vi "Wärmepumpe.ParameterUI.vi"() -> ()   [LabVIEW 2016, in "Wärmepumpe.lvclass"]
uses:
  Package ResourceControl/ViHandler/ViHandler.ViInfo.ctl
  Package Libraries/Message Queue/private/MessageQueue.MessageTypeDef.ctl
  Package ErrorHandling/ErrorHandling.lvclass/ErrorHandling.ctl
  Package ErrorHandling/ErrorHandling.checkForErrorAndHandle.vi
  Package ErrorHandling/ErrorHandling.GetErrorHandler.vi
  Package Libraries/StringFunctions/StringFunctions_ReplaceAllBlindSigns.vi
  <vilib>/dlg_ctls.llb/Space Constant.vi
  <vilib>/Utility/error.llb/Error Cluster From Error Code.vi
  Package Libraries/TimingFunctions/TimingFunctions_getUtcTimestamp.vi
  <vilib>/Utility/error.llb/Trim Whitespace.vi
  <vilib>/Utility/error.llb/Search and Replace Pattern.vi
  Package ErrorHandling/ErrorHandling.addLastErrorToFile.vi
  <vilib>/ErrorRing/Error Ring.xnode
  Package ErrorHandling/ErrorHandling.lvclass
  Package ResourceControl/ViHandler/ViHandler.lvclass
panel:
  in  "Wärmepumpe Parameter":T1
  out "Y-AxisCopy":dbl[](array[numeric])=[54400.0, 48000.0, 40000.0, 30000.0] caption="Y-Axis"
  out "X-AxisCopy":dbl[](array[numeric])=[54400.0, 48000.0, 40000.0, 30000.0] caption="X-Axis"
  in  "Heizleistung":dbl[][](array[numeric])=[[54400.0, 48000.0, 40000.0, 30000.0], [65800.0, 58800.0, 52800.0, 45000.0], [78600.0, 70400.0, 63800.0, 58200.0], [92400.0, 83200.0, 76400.0, 71400.0], [108800.0, 98000.0, 89800.0, 82200.0], [126800.0, 114600.0, 105200.0, 98400.0]]
  out "Y-Axis":dbl[](array[numeric])=[54400.0, 48000.0, 40000.0, 30000.0]
  out "X-Axis":dbl[](array[numeric])=[54400.0, 48000.0, 40000.0, 30000.0]
  in  "Kältelteistung":dbl[][](array[numeric])=[[54400.0, 48000.0, 40000.0, 30000.0], [65800.0, 58800.0, 52800.0, 45000.0], [78600.0, 70400.0, 63800.0, 58200.0], [92400.0, 83200.0, 76400.0, 71400.0], [108800.0, 98000.0, 89800.0, 82200.0], [126800.0, 114600.0, 105200.0, 98400.0]]
  in  "LoadDefBtn":bool
  in  "Model Path":path
  out "Wärmepumpe":refnum<data-value>
  out "ViInfoTemp":T2
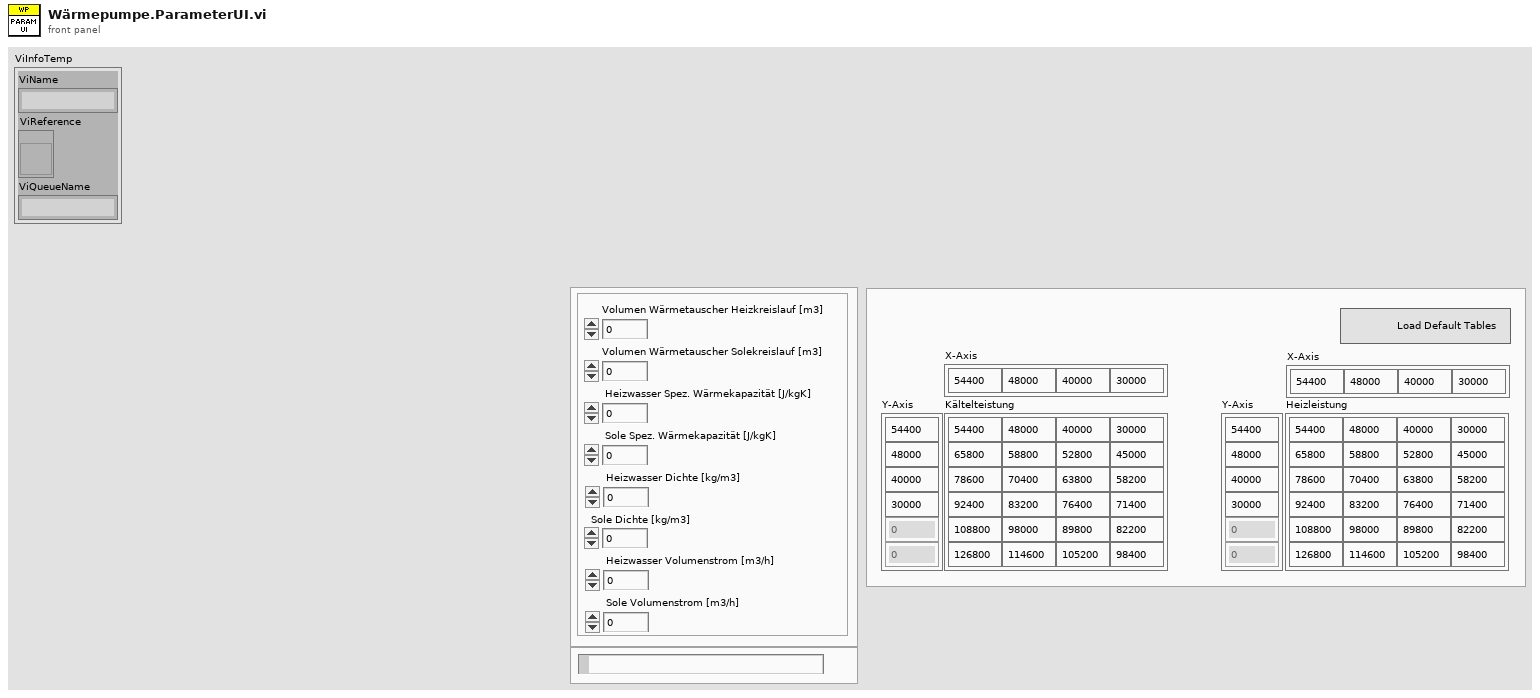
[diagram p1: front panel]
types:
  T1 = cluster{"Volumen Wärmetauscher Heizkreislauf [m3]":dbl, "Volumen Wärmetauscher Solekreislauf [m3]":dbl, " Heizwasser Spez. Wärmekapazität [J/kgK]":dbl, " Sole Spez. Wärmekapazität [J/kgK]":dbl, " Heizwasser Dichte [kg/m3]":dbl, "Sole Dichte [kg/m3] ":dbl, " Heizwasser Volumenstrom [m3/h]":dbl, " Sole Volumenstrom [m3/h]":dbl}
  T2 = typedef "ViHandler.lvclass/ViHandler.ViInfo.ctl" = cluster{"ViName":string, "ViReference":refnum<vi>, "ViQueueName":string}
  T3 = typedef "MessageQueue.MessageTypeDef.ctl" = cluster{"Message":string, "Data":variant}
  T4 = enum16{"open", "replace", "create", "open or create", "replace or create", "replace or create with confirmation"}
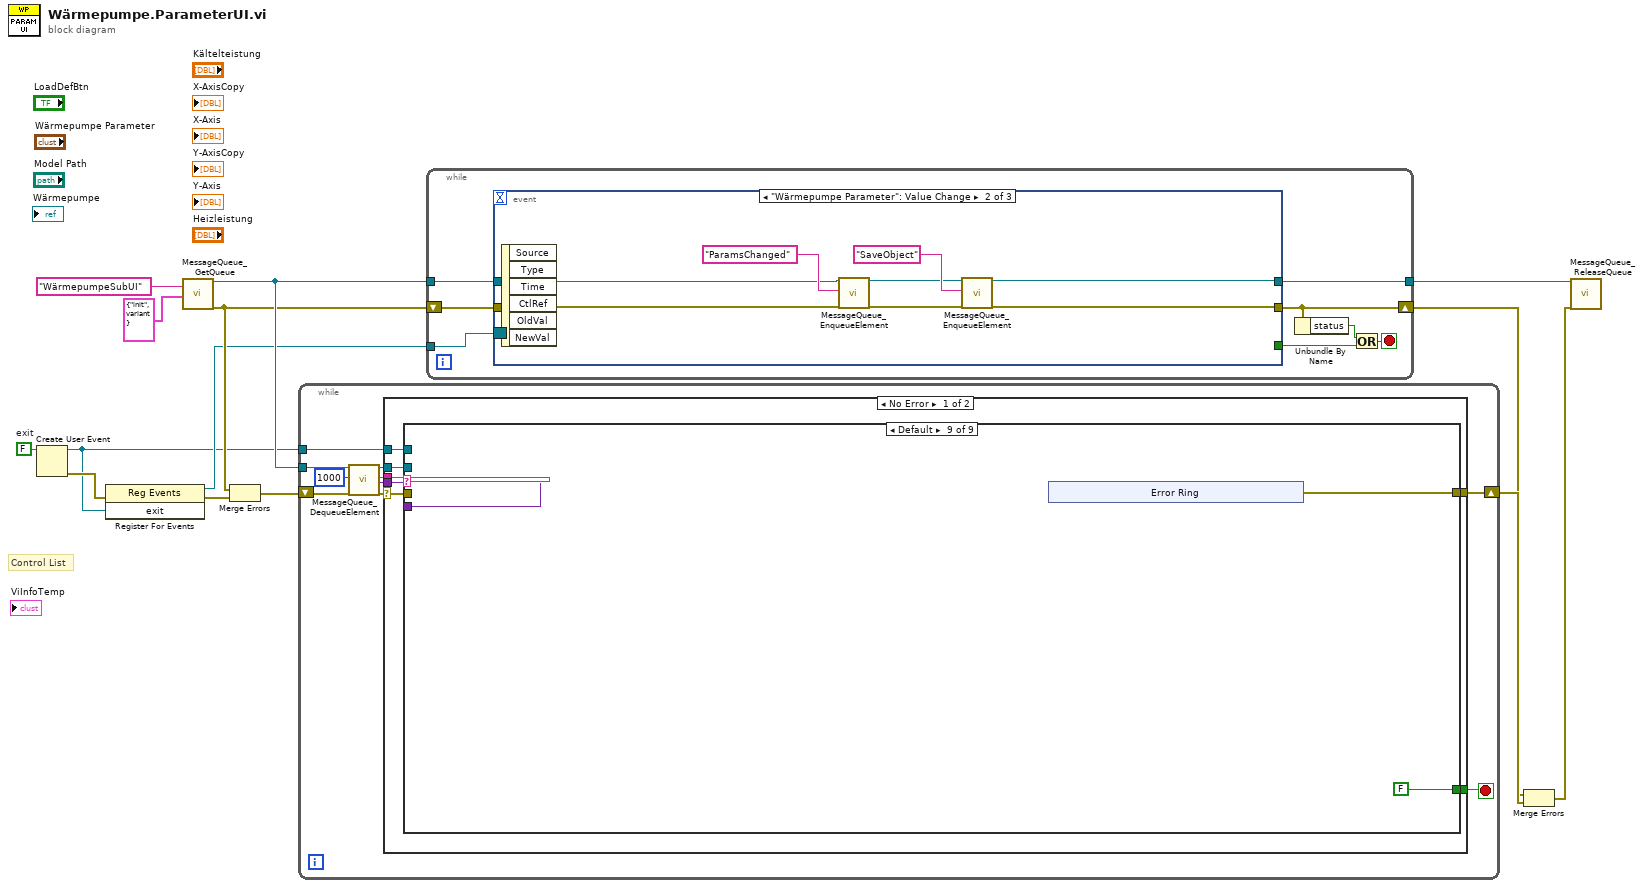
[diagram p0: block diagram]
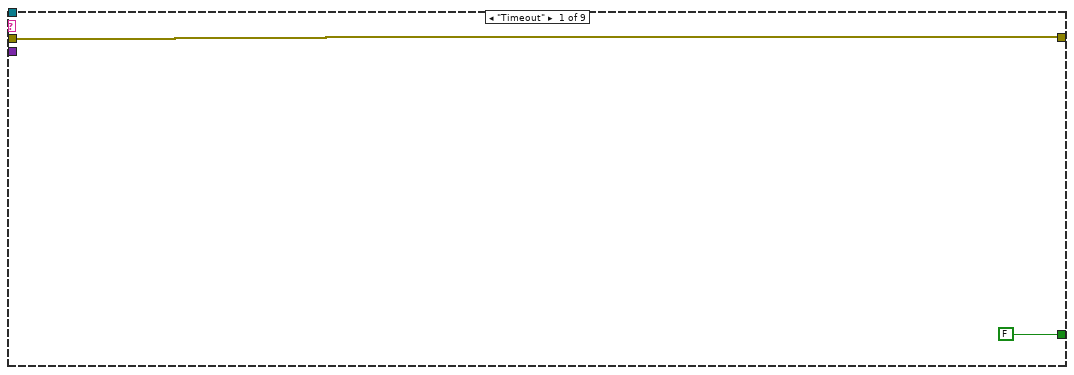
[diagram p2: hidden frame]
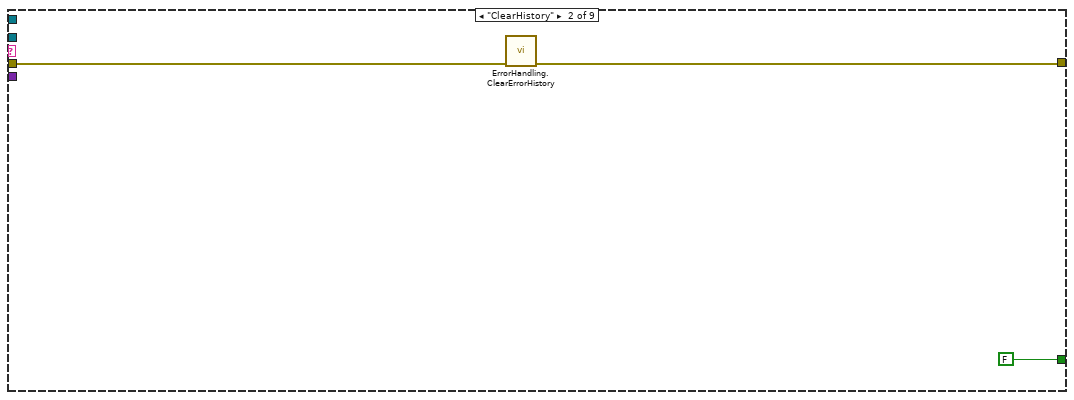
[diagram p3: hidden frame]
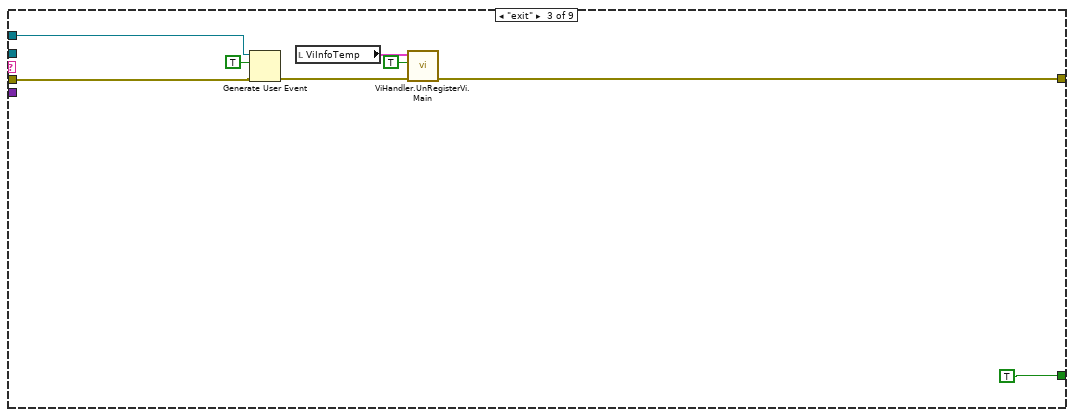
[diagram p4: hidden frame]
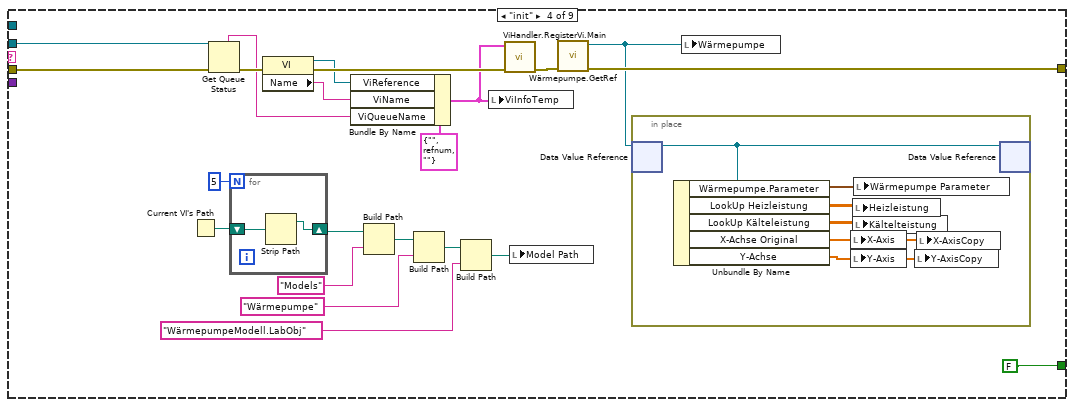
[diagram p5: hidden frame]
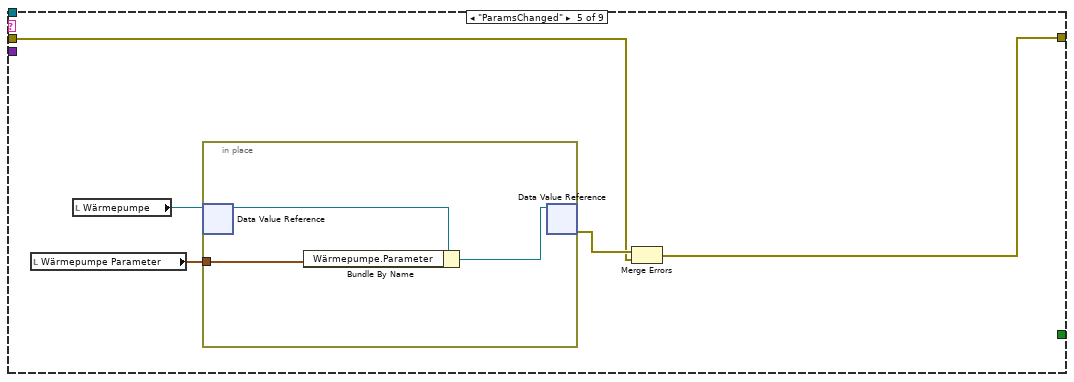
[diagram p6: hidden frame]
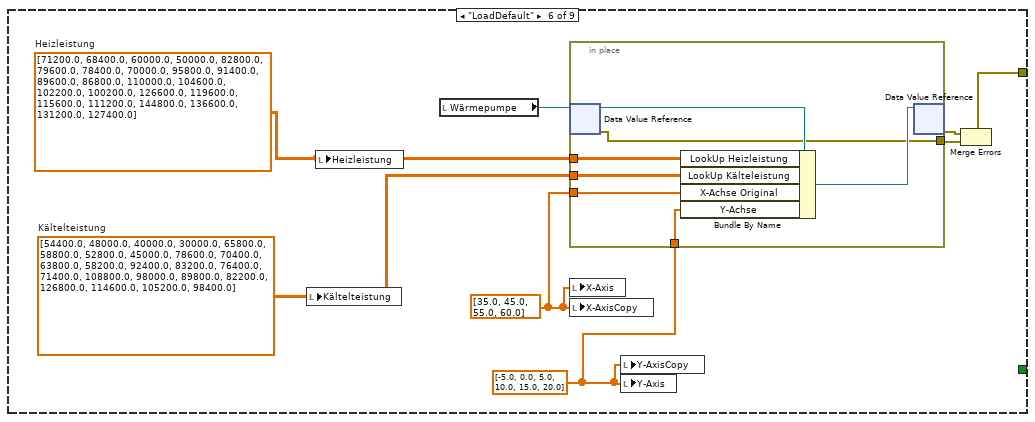
[diagram p7: hidden frame]
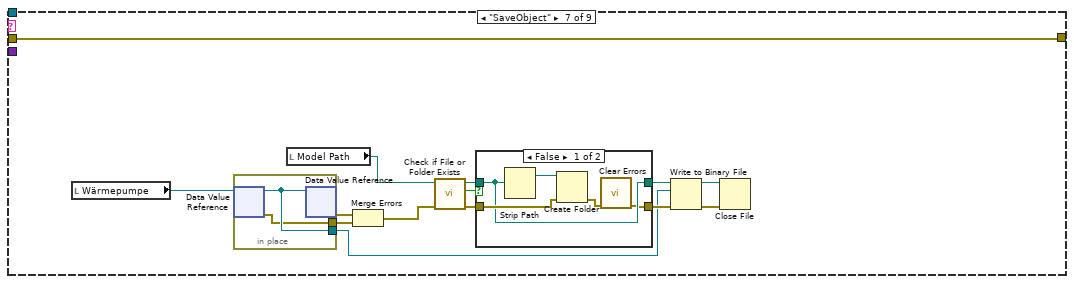
[diagram p8: hidden frame]
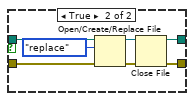
[diagram p9: hidden frame]
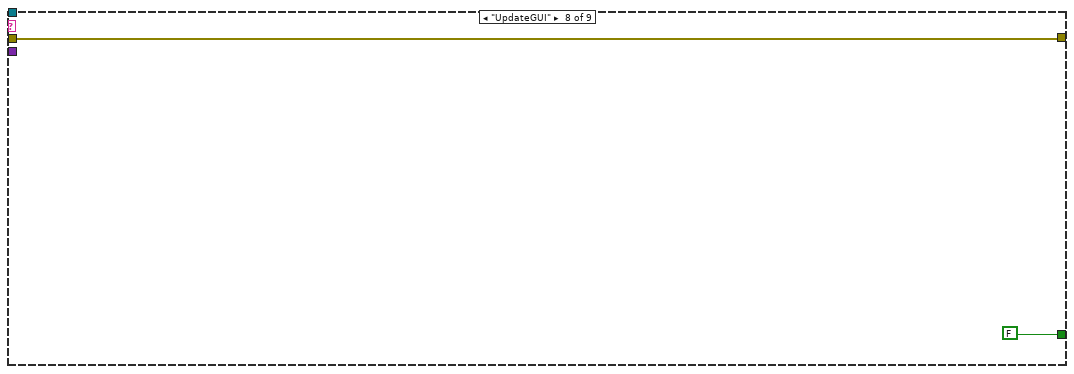
[diagram p10: hidden frame]
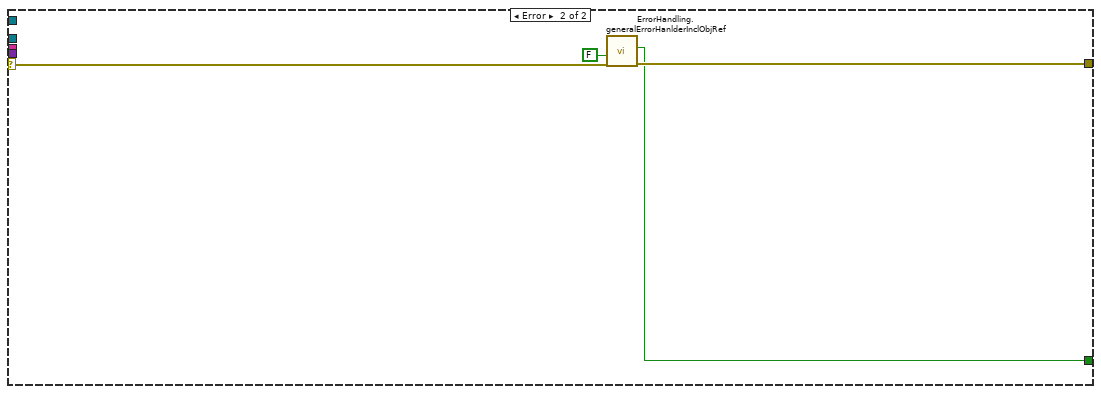
[diagram p11: hidden frame]
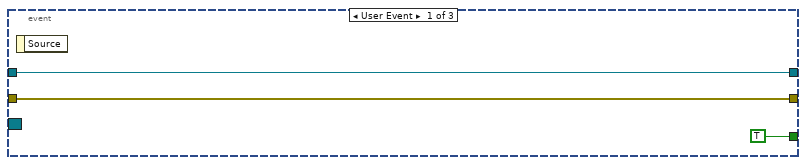
[diagram p12: hidden frame]
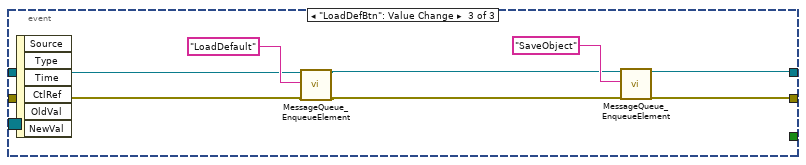
[diagram p13: hidden frame]
diagram:
  w7 = FALSE  # exit
  # "Control List"
  n1 = Create User Event(user event datatype=w7) -> (user event=w5:refnum<user-event>, error out=w6:errorcluster)  [unwired: 1 in]
  n2 = register-events(error in=w6, w5) -> (reference out=w9:refnum<event-registration>, error out=w11:errorcluster)  [unwired: 1 in]
  n3 = call "MessageQueue_GetQueue.vi"("Name"="WärmepumpeSubUI", "OptionalInitValue"=T3 {"Message"="init", "Data"=variant}) -> ("QueueOut"=w13:refnum<queue>, "ErrorOut"=w10:errorcluster)  [unwired: 15 in, 1 out]
  n4 = Merge Errors(w10, w11) -> (w8:errorcluster)
  n5 = while {
    tunnel: w13 -> [w24]
    tunnel: w5 -> [w17]
    shift-right: [w16] -> w3
    shift-left: w8 -> [w18]
    stop <- w19 stop-if-true
    n6 = call "MessageQueue_DequeueElement.vi"("QueueIn"=w24, "Timeout"=1000, "ErrorIn"=w18) -> ("QueueOut"=w22:refnum<queue>, "Message"=w21:string, "Data"=w20:variant, "ErrorOut"=w23:errorcluster)  [unwired: 12 in, 1 out]
    n7 = case shown="No Error" w23 {
      selector: w23 -> [w27 w138]
      tunnel: w22 -> [w31 _]
      tunnel: w21 -> [w30 _]
      tunnel: w20 -> [w29 _]
      tunnel: [w28 w136] -> w19
      tunnel: w17 -> [w26 _]
      tunnel: [w25 w137] -> w16
      frame No Error {
        n8 = case shown="Default" w30 {
          tunnel: w31 -> [_ _ _ w60 _ _ _ _ _]
          tunnel: w29 -> [_ _ _ _ _ _ _ _ _]
          tunnel: [FALSE FALSE TRUE FALSE _ _ _ FALSE FALSE] -> w28
          tunnel: w27 -> [w32 w35 w42 w57 w75 _ w111 w126 _]
          tunnel: w26 -> [_ _ w41 _ _ _ _ _ _]
          tunnel: [w32 w34 w38 w55 w76 w88 w111 w126 w129] -> w25
          frame "Timeout" {
          }
          frame "ClearHistory" {
            n9 = call "ErrorHandling.ClearErrorHistory.vi"("error IO"=w35) -> ("error IO"=w34:errorcluster)  [unwired: 10 in]
          }
          frame "exit" {
            n10 = Generate User Event(user event=w41, event data cluster=TRUE ("event data"), error in=w42) -> (error out=w39:errorcluster)  [unwired: 1 in, 1 out]
            n11 = local read "ViInfoTemp"() -> (w40:T2)
            n12 = call "ViHandler.UnRegisterVi.Main.vi"("ErrorIn"=w39, "FinalExit?"=TRUE, "ViInfo"=w40) -> ("ErrorOut"=w38:errorcluster)  [unwired: 7 in, 1 out]
          }
          frame "init" {
            n13 = Current VI's Path() -> (path=w46:path)
            n14 = Get Queue Status(queue=w60, error in (no error)=w57) -> (queue name=w58:string, error out=w64:errorcluster)  [unwired: 1 in, 6 out]
            n15 = for {
              N: 5 -> [_]
              shift-right: [w73] -> w53
              shift-left: w46 -> [w74]
              n16 = Strip Path(path=w74) -> (stripped path=w73:path)  [unwired: 1 out]
            }
            n17 = property class="VI"(error in=w64) -> (reference out=w62:refnum<vi>, error out=w63:errorcluster, "Name"=w61:string)  [unwired: 1 in]
            n18 = Bundle By Name(cluster=T2 {"ViName"="", "ViReference"=refnum, "ViQueueName"=""} ("ViInfo"), "ViReference"=w62, "ViName"=w61, "ViQueueName"=w58) -> (w59:T2)
            n19 = Build Path(base path=w53, name or relative path="Models") -> (appended path=w51:path)
            n20 = Build Path(base path=w51, name or relative path="Wärmepumpe") -> (appended path=w49:path)
            n21 = Build Path(base path=w49, name or relative path="WärmepumpeModell.LabObj") -> (appended path=w48:path)
            n22 = local write "ViInfoTemp"(w59) -> ()
            n23 = call "ViHandler.RegisterVi.Main.vi"("ErrorIn"=w63, "ViInfo"=w59) -> ("ErrorOut"=w56:errorcluster)  [unwired: 9 in]
            n24 = local write "Model Path"(w48) -> ()
            n25 = call "Wärmepumpe.GetRef.vi"("Error In"=w56) -> ("Error out"=w55:errorcluster, "Wärmepumpe"=w45:refnum<data-value>)  [unwired: 9 in]
            n26 = in-place {
              n27 = in-place-dvr #1(w45) -> (w72:refnum<class "Wärmepumpe.lvclass">)  [unwired: 1 out]
              n28 = Unbundle By Name(w72) -> ("Wärmepumpe.Parameter"=w71:T1, "LookUp Heizleistung"=w70:dbl[][], "LookUp Kälteleistung"=w69:dbl[][], "X-Achse Original"=w68:dbl[], "Y-Achse"=w67:dbl[])
              n29 = local write "X-Axis"(w68) -> ()
              n30 = local write "Y-Axis"(w67) -> ()
              n31 = local write "Heizleistung"(w70) -> ()
              n32 = local write "Kältelteistung"(w69) -> ()
              n33 = local write "Wärmepumpe Parameter"(w71) -> ()
              n34 = local write "Y-AxisCopy"(w67) -> ()
              n35 = local write "X-AxisCopy"(w68) -> ()
              n36 = in-place-dvr #1(w72) -> ()  [unwired: 2 out]
            }
            n37 = local write "Wärmepumpe"(w45) -> ()
          }
          frame "ParamsChanged" {
            n38 = local read "Wärmepumpe Parameter"() -> (w79:T1)
            n39 = local read "Wärmepumpe"() -> (w77:refnum<data-value>)
            n40 = in-place {
              in-place-border: w79 -> [w82]
              n41 = in-place-dvr #2(w77) -> (w81:refnum<class "Wärmepumpe.lvclass">)  [unwired: 1 out]
              n42 = Bundle By Name(cluster=w81, "Wärmepumpe.Parameter"=w82) -> (w80:refnum<class "Wärmepumpe.lvclass">)
              n43 = in-place-dvr #2(w80) -> (w78:errorcluster)  [unwired: 1 out]
            }
            n44 = Merge Errors(w78, w75) -> (w76:errorcluster)
          }
          frame "LoadDefault" {
            w84 = dbl[] [-5.0, 0.0, 5.0, 10.0, 15.0, 20.0]
            w85 = dbl[] [35.0, 45.0, 55.0, 60.0]
            w86 = dbl[][] [[54400.0, 48000.0, 40000.0, 30000.0], [65800.0, 58800.0, 52800.0, 45000.0], [78600.0, 70400.0, 63800.0, 58200.0], [92400.0, 83200.0, 76400.0, 71400.0], [108800.0, 98000.0, 89800.0, 82200.0], [126800.0, 114600.0, 105200.0, 98400.0]]  # Kältelteistung
            w83 = dbl[][] [[71200.0, 68400.0, 60000.0, 50000.0], [82800.0, 79600.0, 78400.0, 70000.0], [95800.0, 91400.0, 89600.0, 86800.0], [110000.0, 104600.0, 102200.0, 100200.0], [126600.0, 119600.0, 115600.0, 111200.0], [144800.0, 136600.0, 131200.0, 127400.0]]  # Heizleistung
            n45 = local write "Kältelteistung"(w86) -> ()
            n46 = local write "Heizleistung"(w83) -> ()
            n47 = local read "Wärmepumpe"() -> (w89:refnum<data-value>)
            n48 = in-place {
              in-place-border: [w95] -> w87
              in-place-border: w85 -> [w94]
              in-place-border: w84 -> [w93]
              in-place-border: w86 -> [w92]
              in-place-border: w83 -> [w91]
              n49 = in-place-dvr #3(w89) -> (w97:refnum<class "Wärmepumpe.lvclass">, w95:errorcluster)
              n50 = Bundle By Name(cluster=w97, "LookUp Heizleistung"=w91, "LookUp Kälteleistung"=w92, "X-Achse Original"=w94, "Y-Achse"=w93) -> (w96:refnum<class "Wärmepumpe.lvclass">)
              n51 = in-place-dvr #3(w96) -> (w90:errorcluster)  [unwired: 1 out]
            }
            n52 = local write "X-Axis"(w85) -> ()
            n53 = local write "X-AxisCopy"(w85) -> ()
            n54 = local write "Y-AxisCopy"(w84) -> ()
            n55 = local write "Y-Axis"(w84) -> ()
            n56 = Merge Errors(w90, w87) -> (w88:errorcluster)
          }
          frame "SaveObject" {
            n57 = local read "Wärmepumpe"() -> (w98:refnum<data-value>)
            n58 = in-place {
              in-place-border: [w113] -> w99
              in-place-border: [w112] -> w103
              n59 = in-place-dvr #4(w98) -> (w113:refnum<class "Wärmepumpe.lvclass">, w112:errorcluster)
              n60 = in-place-dvr #4(w113) -> (w102:errorcluster)  [unwired: 1 out]
            }
            n61 = local read "Model Path"() -> (w100:path)
            n62 = Merge Errors(w102, w103) -> (w101:errorcluster)
            n63 = call <vilib>:"Check if File or Folder Exists.vi"("error in (no error)"=w101, "path"=w100) -> ("error out"=w108:errorcluster, "file or folder exists?"=w110:bool, "dup path"=w109:path)  [unwired: 7 in]
            n64 = case shown="False" w110 {
              tunnel: w109 -> [w116 w125]
              tunnel: [w116 w121] -> w107
              tunnel: w108 -> [w117 w124]
              tunnel: [w114 w120] -> w106
              frame False {
                n65 = Strip Path(path=w116) -> (stripped path=w118:path)  [unwired: 1 out]
                n66 = Create Folder(path (use dialog)=w118, error in=w117) -> (error out=w115:errorcluster)  [unwired: 1 in, 2 out]
                n67 = call <vilib>:"Clear Errors.vi"("error in (no error)"=w115) -> ("error out"=w114:errorcluster)  [unwired: 5 in, 1 out]
              }
              frame True {
                n68 = Open/Create/Replace File(file path (use dialog)=w125, error in=w124, operation (0:open)=T4."replace") -> (refnum out=w122:refnum<file>, error out=w119:errorcluster)  [unwired: 3 in, 1 out]
                n69 = Close File(refnum=w122, error in=w119) -> (path=w121:path, error out=w120:errorcluster)
              }
            }
            n70 = Write to Binary File(file (use dialog)=w107, data=w99, error in=w106) -> (refnum out=w104:refnum<file>, error out=w105:errorcluster)  [unwired: 3 in, 1 out]
            n71 = Close File(refnum=w104, error in=w105) -> ()  [unwired: 2 out]
          }
          frame "UpdateGUI" {
          }
          frame Default {
            n72 = xnode "Error Ring"() -> ("error out"=w129:errorcluster)
          }
        }
      }
      frame Error {
        n73 = call "ErrorHandling.generalErrorHanlderInclObjRef.vi"("error in"=w138, "StopOnError"=FALSE) -> ("error out"=w137:errorcluster, "Stop"=w136:bool)  [unwired: 7 in, 1 out]
      }
    }
  }
  n74 = while {
    tunnel: w13 -> [w146]
    tunnel: [w145] -> w14
    shift-right: [w142] -> w2
    shift-left: w10 -> [w144]
    tunnel: w9 -> [w139]
    stop <- w141 stop-if-true
    n75 = event shown="[1] \"Wärmepumpe Parameter\": Value Change" {
      selector: w139 -> [_ _ _]
      dyn-events: _ -> [_ _ _]
      timeout: _ -> [_ _ _]
      tunnel: w146 -> [w148 w153 w161]
      tunnel: [w148 w152 w164] -> w145
      tunnel: [w147 w151 w163] -> w142
      tunnel: w144 -> [w147 w150 w160]
      tunnel: [TRUE _ _] -> w143
      event User Event {
        n76 = event-data() -> ()  [unwired: 1 in, 1 out]
      }
      event "Wärmepumpe Parameter": Value Change {
        n77 = event-data() -> ()  [unwired: 1 in, 6 out]
        n78 = call "MessageQueue_EnqueueElement.vi"("QueueIn"=w153, "Message"="ParamsChanged", "ErrorIn"=w150) -> ("QueueOut"=w155:refnum<queue>, "ErrorOut"=w154:errorcluster)  [unwired: 15 in]
        n79 = call "MessageQueue_EnqueueElement.vi"("QueueIn"=w155, "Message"="SaveObject", "ErrorIn"=w154) -> ("QueueOut"=w152:refnum<queue>, "ErrorOut"=w151:errorcluster)  [unwired: 15 in]
      }
      event "LoadDefBtn": Value Change {
        n80 = event-data() -> ()  [unwired: 1 in, 6 out]
        n81 = call "MessageQueue_EnqueueElement.vi"("QueueIn"=w161, "Message"="LoadDefault", "ErrorIn"=w160) -> ("QueueOut"=w159:refnum<queue>, "ErrorOut"=w158:errorcluster)  [unwired: 15 in]
        n82 = call "MessageQueue_EnqueueElement.vi"("QueueIn"=w159, "Message"="SaveObject", "ErrorIn"=w158) -> ("QueueOut"=w164:refnum<queue>, "ErrorOut"=w163:errorcluster)  [unwired: 15 in]
      }
    }
    n83 = Unbundle By Name(w142) -> ("status"=w140:bool)
    n84 = Or(x=w140, y=w143) -> (x .or. y?=w141:bool)
  }
  n85 = Merge Errors(w2, w3) -> (w1:errorcluster)
  n86 = call "MessageQueue_ReleaseQueue.vi"("QueueIn"=w14, "ErrorIn"=w1) -> ()  [unwired: 15 in, 3 out]
